vi "ver1(FPGA)_7_8_2013.vi"() -> ()   [LabVIEW 2012]
uses:
  <vilib>/Platform/TimedLoop/XDataNode/timing_clust.ctl
  <vilib>/Platform/TimedLoop/XDataNode/nitl_modes.ctl
  <vilib>/Platform/TimedLoop/XDataNode/wakeup.ctl
  <vilib>/rvi/eio/common/nirviEmuTemplateMethod_errors.vi
  <vilib>/rvi/Emulation/niFpgaSctlEmulationRegisterWithScheduler.vi
  <vilib>/rvi/Emulation/niFpgaSctlEmulationScheduler.vi
  <vilib>/Platform/TimedLoop/XDataNode/XDataNode.xnode
  <vilib>/eio/EIONode/EIONode.xnode
  <vilib>/Platform/TimedLoop/XDataNode/XDNodeRunTimeDep.lvlib
panel:
  in  "Output":bool
  in  "Low Mass Limit":i64
  in  "High Mass Limit":i64
  out "Filter 1 Detector 1 Correlation":i32
  out "Filter 1 Detector 3 Correlation":i32
  out "Velocity Count 1":i32
  in  "Filter 2 threshold":i32=1000
  out "Filter 2 Detector 1 Correlation":i32
  out "Filter 2 Detector 3 Correlation":i32
  out "Velocity Count 2":i32
  in  "Filter 1 threshold":i32=1000
  in  "Filter 3 threshold":i32=1000
  out "Filter 3 Detector 1 Correlation":i32
  out "Filter 3 Detector 3 Correlation":i32
  out "Velocity Count 3":i32
  in  "Filter 4 threshold":i32=1000
  out "Filter 4 Detector 1 Correlation":i32
  out "Filter 4 Detector 3 Correlation":i32
  out "Velocity Count 4":i32
  in  "Filter 5 threshold":i32
  out "Filter 5 Detector 1 Correlation":i32
  out "Filter 5 Detector 3 Correlation":i32
  out "Velocity Count 5":i32
  in  "Filter 6 threshold":i32
  out "Filter 6 Detector 1 Correlation":i32
  out "Filter 6 Detector 3 Correlation":i32
  out "Velocity Count 6":i32
  in  "Filter 7 threshold":i32
  out "Filter 7 Detector 1 Correlation":i32
  out "Filter 7 Detector 3 Correlation":i32
  out "Velocity Count 7":i32
  in  "Noise Level":i32
  out "High Correlation 1":i32
  out "High Correlation 2":i32
  out "High Correlation 3":i32
  out "High Correlation 4":i32
  out "High Correlation 5":i32
  out "High Correlation 6":i32
  out "High Correlation 7":i32
  out "Measured Charge 1":i32
  out "Measured Charge 2":i32
  out "Measured Charge 3":i32
  out "Measured Charge 4":i32
  out "Measured Charge 5":i32
  out "Measured Charge 6":i32
  out "Measured Charge 7":i32
  out "Average 1":i32
  out "Average 2":i32
  out "Average 3":i32
  out "Average 4":i32
  out "Average 5":i32
  out "Average 6":i32
  out "Average 7":i32
  out "Average Out":i32
  in  "Reset Measured Quantities":bool
  out "High Average":i32
  out "High Sample":i32
  out "High Sample I16":i16
  out "Current State 1":u16
  out "Current State 2":u16
  out "Current State 3":u16
  out "Current State 4":u16
  out "Current State 5":u16
  out "Current State 6":u16
  out "Current State 7":u16
  out "Counter 1":i32
  out "Counter 2":i32
  out "Counter 3":i32
  out "Counter 4":i32
  out "Counter 5":i32
  out "Counter 6":i32
  out "Counter 7":i32
  out "Plates":bool
  in  "High Charge Limit":i16
  in  "Low Charge Limit":i16
  in  "High Velocity Count":i32
  in  "Low Velocity Count":i32
  out "Measured Velocity 1":i32
  out "Measured Velocity 2":i32
  out "Measured Velocity 3":i32
  out "Measured Velocity 4":i32
  out "Measured Velocity 5":i32
  out "Measured Velocity 6":i32
  out "Measured Velocity 7":i32
  out "Numeric":i32
  out "IO Module\\AI 0":i16
  out "IO Module\\AI 1":i16
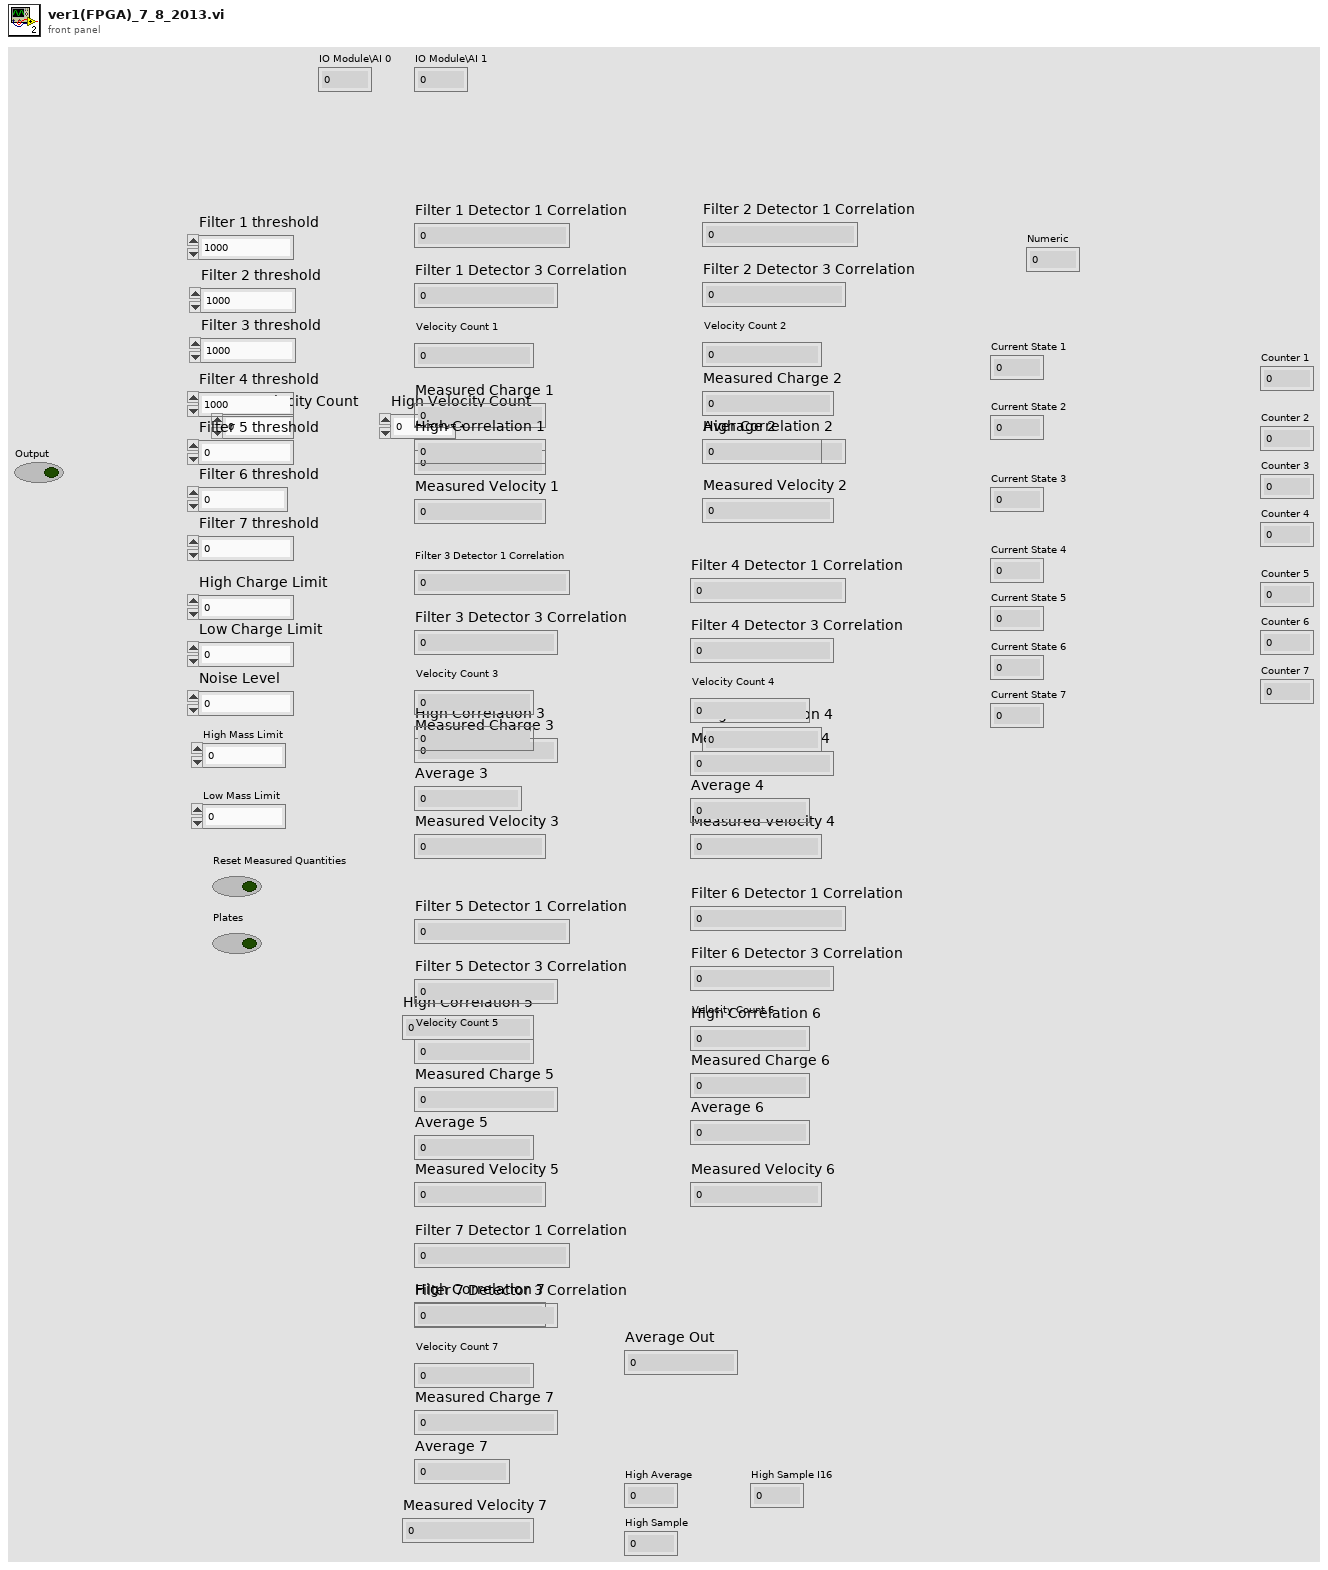
[diagram p1: front panel]
types:
  T1 = typedef "XDNodeRunTimeDep.lvlib/timing_clust.ctl" = cluster{"Expected End [f-1]":u64, "Actual End [f-1]":u64, "Finished Late? [f-1]":bool, "Expected End [i-1]":u64, "Actual End [i-1]":u64, "Finished Late? [i-1]":bool, "Expected Start [i]":u64, "Actual Start [i]":u64, "Expected Start [f]":u64, "Actual Start [f]":u64, "Source Name":string, "Structure Name":string, "Period":i64, "Deadline":i64, "Offset":i64, "Start":i64, "Priority":i32, "Timeout":i32, "Mode":T2, "Wakeup Reason":T3, "Error":errorcluster, "Source Type":string, "Secondary Source Type":string, "Global End Time":u64, "Global Start Time":u64, "Frame Duration":u64, "Iteration Duration":u64, "Assigned CPU":i32, "I/O Scan Engine Mode":u32}
  T2 = typedef "XDNodeRunTimeDep.lvlib/nitl_modes.ctl" = enum32{"No Change", "Process missed periods, maintain original phase", "Discard missed periods, maintain original phase", "Process missed periods, ignore original phase", "Discard missed periods, ignore original phase"}
  T3 = typedef "XDNodeRunTimeDep.lvlib/wakeup.ctl" = enum32{"Normal", "Aborted", "Asynchronous wakeup", "Timing source error", "Timed loop error", "Timeout"}
  T4 = cluster{"Old Average":i32, "New Average":i32, "Current State":u8, "Detector 1 Correlation":i32, "Detector 3 Correlation":i32, "Velocity Count":i32, "Detector Counter in":i32, "Timeout Count in":i32, "Noise Level":i32, "Measured Charge in":i32, "Filter Threshold":i32, "High Correlation in":i32, "Offset":i32, "Offset Average":i32, "Measured Velocity In":i32}
  T5 = cluster{"Separation cut off 1":i32, "Filter Number":i32, "Separation cut off 2":i32}
  T6 = cluster{"High Charge Limit":i16, "Low Charge Limit":i16, "Low Velocity Count":i32, "High Velocity Count":i32, "Low Velocity Count":i32, fxp<+,30,25>, "High Mass Limit":i64, "Low Mass Limit":i64}
  T7 = cluster{"Average Out":i32, "Next State":u8, "Velocity Count out":i32, "Detector counter out":i32, "Timeout count out":u32, "Measured Charge Out":i32, "High Correlation Out":i32, "Plates":bool, "Offset Out":i32, "Measured Velocity Out":i32}
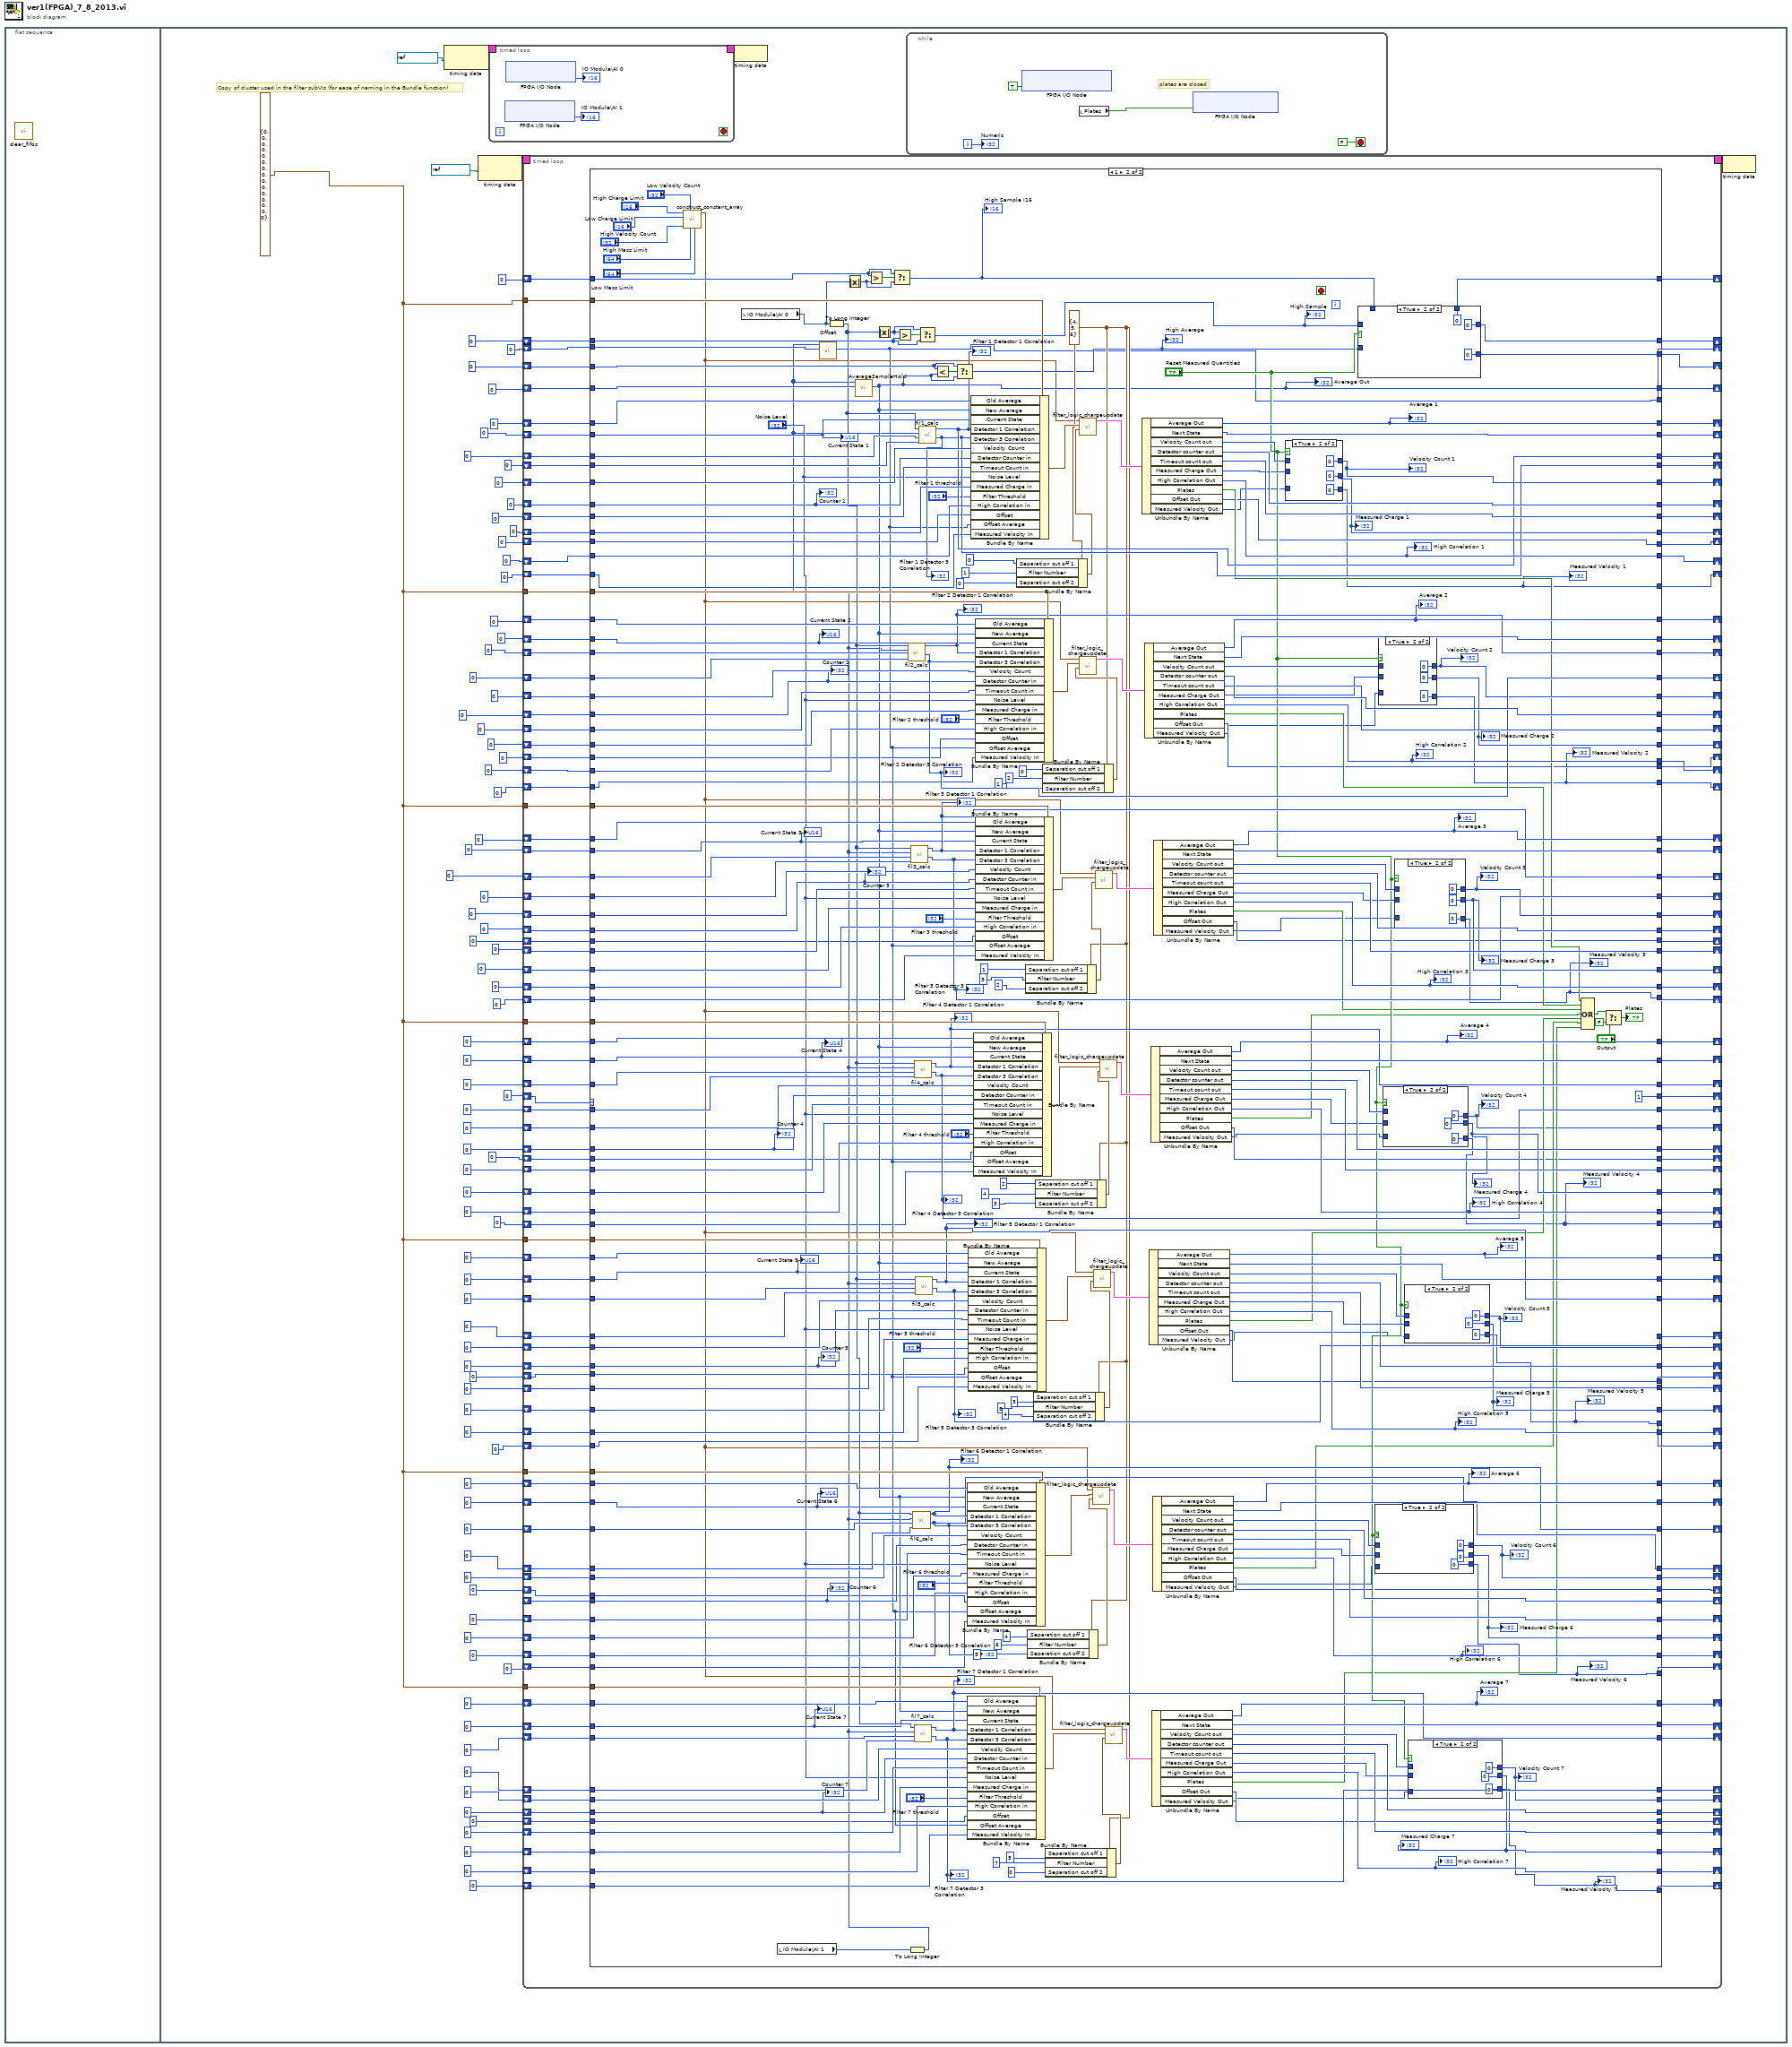
[diagram p0: block diagram]
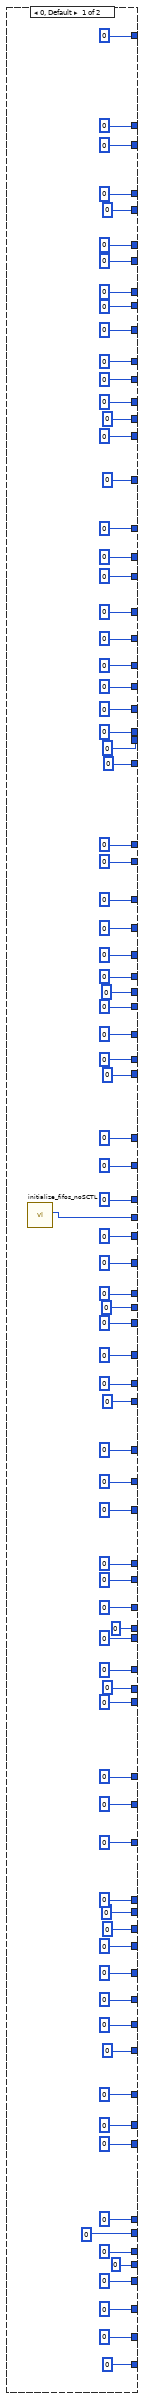
[diagram p2: hidden frame]
diagram:
  n1 = flat-sequence {
    frame #0 {
      n2 = call "clear_fifos.vi"() -> ()  [unwired: 1 in]
    }
    frame #1 {
      w10 = T4 {"Old Average"=0, "New Average"=0, "Current State"=0, "Detector 1 Correlation"=0, "Detector 3 Correlation"=0, "Velocity Count"=0, "Detector Counter in"=0, "Timeout Count in"=0, "Noise Level"=0, "Measured Charge in"=0, "Filter Threshold"=0, "High Correlation in"=0, "Offset"=0, "Offset Average"=0, "Measured Velocity In"=0} ("Variables Cluster")
      # "Copy of cluster used in the filter subVIs (for ease of naming in the Bundle function)"
      n3 = node-c288(refnum<k21> "AI Clock" ("Source Name")) -> (w21:T1)
      n4 = node-c288(refnum<k21> "26 MHz" ("Source Name")) -> (w89:T1)
      n5 = timed-loop {
        timing: w21 -> [_]
        timing-out: [_] -> w20
        stop <- _ stop-if-true
        n6 = xnode "FPGA I/O Node"() -> ("IO Module\\AI 1"=→"IO Module\\AI 1":i16)  [unwired: 1 in, 1 out]
        n7 = xnode "FPGA I/O Node"() -> ("IO Module\\AI 0"=→"IO Module\\AI 0":i16)  [unwired: 1 in, 1 out]
      }
      n8 = timed-loop {
        timing: w89 -> [_]
        timing-out: [_] -> w88
        shift-right: [w267] -> _
        shift-left: 0 ("Velocity Count out") -> [w189]
        shift-right: [w268] -> _
        shift-left: 0 ("Detector 1 Correlation out") -> [w190]
        shift-right: [w154] -> _
        shift-left: 0 ("Detector counter out") -> [w191]
        shift-right: [w185] -> _
        shift-left: 0 ("Next State") -> [w192]
        shift-right: [w153] -> _
        shift-left: 0 ("Detector 3 Correlation out") -> [w188]
        shift-right: [w266] -> _
        shift-left: 0 ("Timeout count out") -> [w187]
        shift-right: [w181] -> _
        shift-left: 0 ("Next State") -> [w184]
        shift-right: [w180] -> _
        shift-left: 0 ("Detector counter out") -> [w183]
        shift-right: [w152] -> _
        shift-left: 0 ("Detector 1 Correlation out") -> [w260]
        shift-right: [w257] -> _
        shift-left: 0 ("Velocity Count out") -> [w259]
        shift-right: [w256] -> _
        shift-left: u32 0 ("Detector 3 Correlation out") -> [w258]
        shift-right: [w251] -> _
        shift-left: 0 ("Timeout count out") -> [w252]
        shift-right: [w175] -> _
        shift-left: 0 ("Next State") -> [w178]
        shift-right: [w150] -> _
        shift-left: 0 ("Detector counter out") -> [w248]
        shift-right: [w246] -> _
        shift-left: 0 ("Detector 1 Correlation out") -> [w247]
        shift-right: [w244] -> _
        shift-left: u32 0 ("Velocity Count out") -> [w245]
        shift-right: [w149] -> _
        shift-left: 0 ("Detector 3 Correlation out") -> [w243]
        shift-right: [w242] -> _
        shift-left: 0 ("Timeout count out") -> [w177]
        shift-right: [w269] -> _
        shift-left: u8 0 ("High Correlation Out") -> [w272]
        shift-right: [w261] -> _
        shift-left: u8 0 ("High Correlation Out") -> [w262]
        shift-right: [w176] -> _
        shift-left: 0 ("High Correlation Out") -> [w179]
        shift-right: [w270] -> _
        shift-left: 0 ("Measured Charge Out") -> [w273]
        shift-right: [w263] -> _
        shift-left: 0 ("Measured Charge Out") -> [w264]
        shift-right: [w250] -> _
        shift-left: u8 0 ("Measured Charge Out") -> [w249]
        shift-right: [w138] -> _
        shift-left: 0 ("Output New Average") -> [w274]
        shift-right: [w186] -> _
        shift-left: 0 ("Detector 1 Correlation Out") -> [w193]
        tunnel: w10 -> [w271]
        shift-right: [w151] -> _
        shift-left: 0 ("High Sample Out") -> [w254]
        shift-right: [w255] -> _
        shift-left: 0 ("High Correlation Out") -> [w182]
        tunnel: w10 -> [w265]
        tunnel: w10 -> [w253]
        shift-right: [w241] -> _
        shift-left: 0 ("Average Out") -> [w240]
        shift-right: [w239] -> _
        shift-left: u8 0 ("Next State") -> [w238]
        shift-right: [w171] -> _
        shift-left: 0 ("Detector 1 Correlation out") -> [w173]
        shift-right: [w170] -> _
        shift-left: 0 ("Detector 3 Correlation out") -> [w172]
        shift-right: [w148] -> _
        shift-left: 0 ("Velocity Count out") -> [w237]
        shift-right: [w236] -> _
        shift-left: 0 ("Detector counter out") -> [w235]
        shift-right: [w234] -> _
        shift-left: u32 0 ("Timeout count out") -> [w233]
        shift-right: [w147] -> _
        shift-left: 0 ("Measured Charge Out") -> [w232]
        shift-right: [w231] -> _
        shift-left: 0 ("High Correlation Out") -> [w174]
        tunnel: w10 -> [w230]
        shift-right: [w228] -> _
        shift-left: 0 ("Average Out") -> [w227]
        shift-right: [w226] -> _
        shift-left: u8 0 ("Next State") -> [w225]
        shift-right: [w166] -> _
        shift-left: 0 ("Detector 1 Correlation out") -> [w169]
        shift-right: [w165] -> _
        shift-left: 0 ("Detector 3 Correlation out") -> [w168]
        shift-right: [w146] -> _
        shift-left: 0 ("Velocity Count out") -> [w224]
        shift-right: [w223] -> _
        shift-left: 0 ("Detector counter out") -> [w222]
        shift-right: [w221] -> _
        shift-left: u32 0 ("Timeout count out") -> [w220]
        shift-right: [w145] -> _
        shift-left: 0 ("Measured Charge Out") -> [w219]
        shift-right: [w218] -> _
        shift-left: 0 ("High Correlation Out") -> [w167]
        tunnel: w10 -> [w229]
        shift-right: [w216] -> _
        shift-left: 0 ("Average Out") -> [w214]
        shift-right: [w215] -> _
        shift-left: u8 0 ("Next State") -> [w211]
        shift-right: [w161] -> _
        shift-left: 0 ("Detector 1 Correlation out") -> [w164]
        shift-right: [w160] -> _
        shift-left: 0 ("Detector 3 Correlation out") -> [w163]
        shift-right: [w143] -> _
        shift-left: 0 ("Velocity Count out") -> [w213]
        shift-right: [w210] -> _
        shift-left: _ -> [w212]
        shift-right: [w209] -> _
        shift-left: u32 0 ("Timeout count out") -> [w208]
        shift-right: [w144] -> _
        shift-left: 0 ("Measured Charge Out") -> [w207]
        shift-right: [w206] -> _
        shift-left: 0 ("High Correlation Out") -> [w162]
        tunnel: w10 -> [w217]
        shift-right: [w204] -> _
        shift-left: 0 ("Average Out") -> [w203]
        shift-right: [w202] -> _
        shift-left: u8 0 ("Next State") -> [w194]
        shift-right: [w156] -> _
        shift-left: 0 ("Detector 1 Correlation out") -> [w159]
        shift-right: [w155] -> _
        shift-left: 0 ("Detector 3 Correlation out") -> [w158]
        shift-right: [w142] -> _
        shift-left: 0 ("Velocity Count out") -> [w201]
        shift-right: [w200] -> _
        shift-left: 0 ("Detector counter out") -> [w199]
        shift-right: [w198] -> _
        shift-left: u32 0 ("Timeout count out") -> [w197]
        shift-right: [w141] -> _
        shift-left: 0 ("Measured Charge Out") -> [w196]
        shift-right: [w195] -> _
        shift-left: 0 ("High Correlation Out") -> [w157]
        tunnel: w10 -> [w205]
        shift-right: [w136] -> _
        shift-left: 0 -> [w137]
        shift-right: [w139] -> _
        shift-left: 0 -> [w140]
        shift-right: [w134] -> _
        shift-left: i16 0 -> [w135]
        shift-right: [w132] -> _
        shift-left: i16 0 -> [w133]
        shift-right: [w130] -> _
        shift-left: 0 -> [w131]
        shift-right: [w129] -> _
        shift-left: 0 -> [w126]
        shift-right: [w127] -> _
        shift-left: 0 -> [w128]
        shift-right: [w124] -> _
        shift-left: 0 ("Offset Out") -> [w125]
        shift-right: [w123] -> _
        shift-left: 0 ("Offset Out") -> [w122]
        shift-right: [w121] -> _
        shift-left: 0 ("Offset Out") -> [w120]
        shift-right: [w119] -> _
        shift-left: 0 ("Offset Out") -> [w118]
        shift-right: [w117] -> _
        shift-left: 0 ("Offset Out") -> [w116]
        shift-right: [w114] -> _
        shift-left: 0 -> [w115]
        shift-right: [w113] -> _
        shift-left: 0 -> [w102]
        shift-right: [w112] -> _
        shift-left: 0 -> [w103]
        shift-right: [w111] -> _
        shift-left: 0 -> [w104]
        shift-right: [w110] -> _
        shift-left: 0 -> [w105]
        shift-right: [w109] -> _
        shift-left: 0 -> [w106]
        shift-right: [w108] -> _
        shift-left: 0 ("Measured Velocity Out") -> [w107]
        stop <- _ stop-if-true
        n9 = case shown="1" w133 {
          tunnel: w274 -> [_ w632]
          tunnel: w273 -> [_ w631]
          tunnel: w272 -> [_ w424]
          tunnel: w271 -> [_ w630]
          tunnel: [0 ("Average Out") w629] -> w270
          tunnel: [u16 0 ("Next State") w628] -> w269
          tunnel: [0 ("Detector counter out") w627] -> w268
          tunnel: [u32 0 ("Timeout count out") w626] -> w267
          tunnel: [0 ("High Correlation Out") w625] -> w266
          tunnel: w265 -> [_ w624]
          tunnel: w264 -> [_ w623]
          tunnel: [0 ("Average Out") w622] -> w263
          tunnel: w262 -> [_ w423]
          tunnel: [u16 0 ("Next State") w621] -> w261
          tunnel: w260 -> [_ w620]
          tunnel: w259 -> [_ w416]
          tunnel: w258 -> [_ w619]
          tunnel: [0 ("Detector counter out") w618] -> w257
          tunnel: [u32 0 ("Timeout count out") w617] -> w256
          tunnel: [0 ("High Correlation Out") w616] -> w255
          tunnel: w254 -> [_ w615]
          tunnel: w253 -> [_ w614]
          tunnel: w252 -> [_ w613]
          tunnel: [0 ("Average Out") w612] -> w251
          tunnel: [u16 0 ("Next State") w611] -> w250
          tunnel: w249 -> [_ w422]
          tunnel: w248 -> [_ w610]
          tunnel: w247 -> [_ w415]
          tunnel: [0 ("Detector counter out") w609] -> w246
          tunnel: w245 -> [_ w608]
          tunnel: [u32 0 ("Timeout count out") w607] -> w244
          tunnel: w243 -> [_ w606]
          tunnel: [0 ("High Correlation Out") w605] -> w242
          tunnel: [0 ("Average Out") w604] -> w241
          tunnel: w240 -> [_ w603]
          tunnel: [u16 0 ("Next State") w602] -> w239
          tunnel: w238 -> [_ w421]
          tunnel: w237 -> [_ w601]
          tunnel: [0 ("Detector counter out") w600] -> w236
          tunnel: w235 -> [_ w414]
          tunnel: [u32 0 ("Timeout count out") w599] -> w234
          tunnel: w233 -> [_ w598]
          tunnel: w232 -> [_ w597]
          tunnel: [0 ("High Correlation Out") w596] -> w231
          tunnel: w230 -> [_ w595]
          tunnel: w229 -> [_ w594]
          tunnel: [0 ("Average Out") w593] -> w228
          tunnel: w227 -> [_ w592]
          tunnel: [u16 0 ("Next State") w591] -> w226
          tunnel: w225 -> [_ w420]
          tunnel: w224 -> [_ w590]
          tunnel: [0 ("Detector counter out") w589] -> w223
          tunnel: w222 -> [_ w413]
          tunnel: [u32 0 ("Timeout count out") w588] -> w221
          tunnel: w220 -> [_ w587]
          tunnel: w219 -> [_ w586]
          tunnel: [0 ("High Correlation Out") w585] -> w218
          tunnel: w217 -> [_ w584]
          tunnel: [0 ("Average Out") w583] -> w216
          tunnel: [u16 0 ("Next State") w582] -> w215
          tunnel: w214 -> [_ w581]
          tunnel: w213 -> [_ w580]
          tunnel: w212 -> [_ w412]
          tunnel: w211 -> [_ w419]
          tunnel: [0 ("Detector counter out") w579] -> w210
          tunnel: [u32 0 ("Timeout count out") w578] -> w209
          tunnel: w208 -> [_ w577]
          tunnel: w207 -> [_ w576]
          tunnel: [0 ("High Correlation Out") w575] -> w206
          tunnel: w205 -> [_ w574]
          tunnel: [0 ("Average Out") w573] -> w204
          tunnel: w203 -> [_ w572]
          tunnel: [u16 0 ("Next State") w571] -> w202
          tunnel: w201 -> [_ w570]
          tunnel: [0 ("Detector counter out") w569] -> w200
          tunnel: w199 -> [_ w411]
          tunnel: [u32 0 ("Timeout count out") w568] -> w198
          tunnel: w197 -> [_ w567]
          tunnel: w196 -> [_ w566]
          tunnel: [0 ("High Correlation Out") w565] -> w195
          tunnel: w194 -> [_ w418]
          tunnel: w193 -> [_ w564]
          tunnel: w192 -> [_ w563]
          tunnel: w191 -> [_ w562]
          tunnel: w190 -> [_ w417]
          tunnel: w189 -> [_ w561]
          tunnel: w188 -> [_ w560]
          tunnel: w187 -> [_ w559]
          tunnel: [0 ("Detector 1 Correlation Out") w558] -> w186
          tunnel: [0 ("Detector 3 Correlation Out") w557] -> w185
          tunnel: w184 -> [_ w556]
          tunnel: w183 -> [_ w555]
          tunnel: w182 -> [_ w554]
          tunnel: [0 ("Detector 1 Correlation Out") w553] -> w181
          tunnel: [0 ("Detector 3 Correlation Out") w552] -> w180
          tunnel: w179 -> [_ w551]
          tunnel: w178 -> [_ w550]
          tunnel: w177 -> [_ w549]
          tunnel: [0 ("Detector 1 Correlation Out") w548] -> w176
          tunnel: [0 ("Detector 3 Correlation Out") w547] -> w175
          tunnel: w174 -> [_ w546]
          tunnel: w173 -> [_ w545]
          tunnel: w172 -> [_ w544]
          tunnel: [0 ("Detector 1 Correlation Out") w543] -> w171
          tunnel: [0 ("Detector 3 Correlation Out") w542] -> w170
          tunnel: w169 -> [_ w541]
          tunnel: w168 -> [_ w540]
          tunnel: w167 -> [_ w539]
          tunnel: [0 ("Detector 1 Correlation Out") w538] -> w166
          tunnel: [0 ("Detector 3 Correlation Out") w537] -> w165
          tunnel: w164 -> [_ w536]
          tunnel: w163 -> [_ w535]
          tunnel: w162 -> [_ w534]
          tunnel: [0 ("Detector 1 Correlation Out") w533] -> w161
          tunnel: [0 ("Detector 3 Correlation Out") w532] -> w160
          tunnel: w159 -> [_ w531]
          tunnel: w158 -> [_ w530]
          tunnel: w157 -> [_ w529]
          tunnel: [0 ("Detector 1 Correlation Out") w528] -> w156
          tunnel: [0 ("Detector 3 Correlation Out") w527] -> w155
          tunnel: [0 ("Velocity Count out") w526] -> w154
          tunnel: [0 ("Measured Charge Out") w525] -> w153
          tunnel: [0 ("Velocity Count out") w524] -> w152
          tunnel: [0 ("Measured Charge Out") w523] -> w151
          tunnel: [0 ("Velocity Count out") w522] -> w150
          tunnel: [0 ("Measured Charge Out") w521] -> w149
          tunnel: [0 ("Velocity Count out") w410] -> w148
          tunnel: [0 ("Measured Charge Out") w520] -> w147
          tunnel: [0 ("Velocity Count out") w519] -> w146
          tunnel: [0 ("Measured Charge Out") w518] -> w145
          tunnel: [0 ("Measured Charge Out") w517] -> w144
          tunnel: [0 ("Velocity Count out") w516] -> w143
          tunnel: [0 ("Velocity Count out") w515] -> w142
          tunnel: [0 ("Measured Charge Out") w514] -> w141
          tunnel: w140 -> [_ w513]
          tunnel: [0 w512] -> w139
          tunnel: [0 ("Output New Average") w409] -> w138
          tunnel: w137 -> [_ w511]
          tunnel: [0 w510] -> w136
          tunnel: w135 -> [_ w509]
          tunnel: [i16 0 w508] -> w134
          tunnel: [w357 i16 1 ("Output State")] -> w132
          tunnel: w131 -> [_ w406]
          tunnel: [0 ("Offset Out") w405] -> w130
          tunnel: [0 ("Offset Out") w404] -> w129
          tunnel: w128 -> [_ w403]
          tunnel: [0 ("Output New Average") w392] -> w127
          tunnel: w126 -> [_ w401]
          tunnel: w125 -> [_ w400]
          tunnel: [0 ("Offset Out") w399] -> w124
          tunnel: [0 ("Offset Out") w398] -> w123
          tunnel: w122 -> [_ w397]
          tunnel: [0 ("Offset Out") w396] -> w121
          tunnel: w120 -> [_ w395]
          tunnel: [0 ("Offset Out") w394] -> w119
          tunnel: w118 -> [_ w393]
          tunnel: [0 ("Offset Out") w391] -> w117
          tunnel: w116 -> [_ w390]
          tunnel: w115 -> [_ w385]
          tunnel: [0 ("Measured Velocity Out") w377] -> w114
          tunnel: [0 ("Measured Velocity Out") w375] -> w113
          tunnel: [0 ("Measured Velocity Out") w373] -> w112
          tunnel: [0 ("Measured Velocity Out") w371] -> w111
          tunnel: [0 ("Measured Velocity Out") w369] -> w110
          tunnel: [0 ("Measured Velocity Out") w367] -> w109
          tunnel: [0 ("Measured Velocity Out") w365] -> w108
          tunnel: w107 -> [_ w384]
          tunnel: w106 -> [_ w383]
          tunnel: w105 -> [_ w382]
          tunnel: w104 -> [_ w381]
          tunnel: w103 -> [_ w380]
          tunnel: w102 -> [_ w379]
          frame 0, Default {
            n10 = call "initialize_fifos_noSCTL.vi"() -> ("Output State"=w357:i16)  [unwired: 11 in]
          }
          frame 1 {
            w460 = T5 {"Separation cut off 1"=4, "Filter Number"=5, "Separation cut off 2"=6} ("Filter Specific Constants")
            n11 = call "construct_constant_array.vi"("Low Mass Limit"="Low Mass Limit", "High Mass Limit"="High Mass Limit", "Low Velocity Count"="Low Velocity Count", "High Velocity Count"="High Velocity Count", "Low Charge Limit"="Low Charge Limit", "High Charge Limit"="High Charge Limit") -> ("constants cluster"=w362:T6)  [unwired: 5 in]
            n12 = local read "IO Module\\AI 0"() -> (w408:i16)
            n13 = local read "IO Module\\AI 1"() -> (w407:i16)
            n14 = To Long Integer(number=w408) -> (32bit integer=w441:i32)
            n15 = Absolute Value(x=w408) -> (abs(x)=w434:i16)
            n16 = Greater?(x=w509, y=w434) -> (0:w435:bool)
            n17 = Absolute Value(x=w441) -> (abs(x)=w439:i32)
            n18 = Select(t=w509, s=w435, f=w434) -> (s? t:f=w433:i16)
            "High Sample I16" <- w433
            n19 = Greater?(x=w439, y=w513) -> (0:w440:bool)
            n20 = To Long Integer(number=w407) -> (32bit integer=w402:i32)
            n21 = call "Offset.vi"("Previous Average"=w403, "Input Value"=w402) -> ("Output New Average"=w392:i32)  [unwired: 7 in]
            n22 = call "AverageSampleHold.vi"("Previous Average"=w632, "Input Value"=w402) -> ("Output New Average"=w409:i32)  [unwired: 7 in]
            "Average Out" <- w409
            n23 = call "fil2_calc.vi"("Detector 3 Correlation In"=w555, "Detector 1 Correlation In"=w556, "AI1"=w402, "AI0"=w441) -> ("Detector 3 Correlation Out"=w552:i32, "Detector 1 Correlation Out"=w553:i32)  [unwired: 4 in]
            "Filter 2 Detector 1 Correlation" <- w553
            "Filter 2 Detector 3 Correlation" <- w552
            n24 = call "fil3_calc.vi"("Detector 3 Correlation In"=w550, "Detector 1 Correlation In"=w551, "AI1"=w402, "AI0"=w441) -> ("Detector 3 Correlation Out"=w547:i32, "Detector 1 Correlation Out"=w548:i32)  [unwired: 4 in]
            "Filter 3 Detector 1 Correlation" <- w548
            "Filter 3 Detector 3 Correlation" <- w547
            n25 = call "fil6_calc.vi"("Detector 3 Correlation In"=w535, "Detector 1 Correlation In"=w536, "AI1"=w402, "AI0"=w441) -> ("Detector 3 Correlation Out"=w532:i32, "Detector 1 Correlation Out"=w533:i32)  [unwired: 4 in]
            "Filter 6 Detector 1 Correlation" <- w533
            "Filter 6 Detector 3 Correlation" <- w532
            n26 = call "fil4_calc.vi"("Detector 3 Correlation In"=w544, "Detector 1 Correlation In"=w545, "AI1"=w402, "AI0"=w441) -> ("Detector 3 Correlation Out"=w542:i32, "Detector 1 Correlation Out"=w543:i32)  [unwired: 4 in]
            "Filter 4 Detector 1 Correlation" <- w543
            "Filter 4 Detector 3 Correlation" <- w542
            n27 = call "fil7_calc.vi"("Detector 3 Correlation In"=w530, "Detector 1 Correlation In"=w531, "AI1"=w402, "AI0"=w441) -> ("Detector 3 Correlation Out"=w527:i32, "Detector 1 Correlation Out"=w528:i32)  [unwired: 4 in]
            "Filter 7 Detector 1 Correlation" <- w528
            "Filter 7 Detector 3 Correlation" <- w527
            n28 = call "fil5_calc.vi"("Detector 3 Correlation In"=w540, "Detector 1 Correlation In"=w541, "AI1"=w402, "AI0"=w441) -> ("Detector 3 Correlation Out"=w537:i32, "Detector 1 Correlation Out"=w538:i32)  [unwired: 4 in]
            "Filter 5 Detector 1 Correlation" <- w538
            "Filter 5 Detector 3 Correlation" <- w537
            n29 = call "fil1_calc.vi"("Detector 3 Correlation In"=w563, "Detector 1 Correlation In"=w564, "AI1"=w402, "AI0"=w441) -> ("Detector 3 Correlation Out"=w557:i32, "Detector 1 Correlation Out"=w558:i32)  [unwired: 4 in]
            "Filter 1 Detector 1 Correlation" <- w558
            "Filter 1 Detector 3 Correlation" <- w557
            n30 = Select(t=w439, s=w440, f=w513) -> (s? t:f=w436:i32)
            "High Sample" <- w436
            n31 = Less?(x=w511, y=w409) -> (x < y?=w438:bool)
            n32 = Select(t=w511, s=w438, f=w409) -> (s? t:f=w437:i32)
            "High Average" <- w437
            n33 = Bundle By Name(cluster=w584, "Old Average"=w581, "New Average"=w409, "Current State"=w419, "Detector 1 Correlation"=w533, "Detector 3 Correlation"=w532, "Velocity Count"=w580, "Detector Counter in"=w412, "Timeout Count in"=w577, "Noise Level"="Noise Level", "Measured Charge in"=w576, "Filter Threshold"="Filter 6 threshold", "High Correlation in"=w534, "Offset"=w393, "Offset Average"=w392, "Measured Velocity In"=w383) -> (w482:T4)
            n34 = Bundle By Name(cluster=w574, "Old Average"=w572, "New Average"=w409, "Current State"=w418, "Detector 1 Correlation"=w528, "Detector 3 Correlation"=w527, "Velocity Count"=w570, "Detector Counter in"=w411, "Timeout Count in"=w567, "Noise Level"="Noise Level", "Measured Charge in"=w566, "Filter Threshold"="Filter 7 threshold", "High Correlation in"=w529, "Offset"=w390, "Offset Average"=w392, "Measured Velocity In"=w384) -> (w497:T4)
            n35 = Bundle By Name(cluster=w594, "Old Average"=w592, "New Average"=w409, "Current State"=w420, "Detector 1 Correlation"=w538, "Detector 3 Correlation"=w537, "Velocity Count"=w590, "Detector Counter in"=w413, "Timeout Count in"=w587, "Noise Level"="Noise Level", "Measured Charge in"=w586, "Filter Threshold"="Filter 5 threshold", "High Correlation in"=w539, "Offset"=w395, "Offset Average"=w392, "Measured Velocity In"=w382) -> (w485:T4)
            n36 = Bundle By Name(cluster=w630, "Old Average"=w631, "New Average"=w409, "Current State"=w424, "Detector 1 Correlation"=w558, "Detector 3 Correlation"=w557, "Velocity Count"=w562, "Detector Counter in"=w417, "Timeout Count in"=w561, "Noise Level"="Noise Level", "Measured Charge in"=w560, "Filter Threshold"="Filter 1 threshold", "High Correlation in"=w559, "Offset"=w406, "Offset Average"=w392, "Measured Velocity In"=w385) -> (w494:T4)
            n37 = Bundle By Name(cluster=w595, "Old Average"=w603, "New Average"=w409, "Current State"=w421, "Detector 1 Correlation"=w543, "Detector 3 Correlation"=w542, "Velocity Count"=w601, "Detector Counter in"=w414, "Timeout Count in"=w598, "Noise Level"="Noise Level", "Measured Charge in"=w597, "Filter Threshold"="Filter 4 threshold", "High Correlation in"=w546, "Offset"=w397, "Offset Average"=w392, "Measured Velocity In"=w381) -> (w488:T4)
            n38 = Bundle By Name(cluster=w624, "Old Average"=w623, "New Average"=w409, "Current State"=w423, "Detector 1 Correlation"=w553, "Detector 3 Correlation"=w552, "Velocity Count"=w620, "Detector Counter in"=w416, "Timeout Count in"=w619, "Noise Level"="Noise Level", "Measured Charge in"=w615, "Filter Threshold"="Filter 2 threshold", "High Correlation in"=w554, "Offset"=w401, "Offset Average"=w392, "Measured Velocity In"=w379) -> (w506:T4)
            n39 = Bundle By Name(cluster=w614, "Old Average"=w613, "New Average"=w409, "Current State"=w422, "Detector 1 Correlation"=w548, "Detector 3 Correlation"=w547, "Velocity Count"=w610, "Detector Counter in"=w415, "Timeout Count in"=w608, "Noise Level"="Noise Level", "Measured Charge in"=w606, "Filter Threshold"="Filter 3 threshold", "High Correlation in"=w549, "Offset"=w400, "Offset Average"=w392, "Measured Velocity In"=w380) -> (w491:T4)
            n40 = Bundle By Name(cluster=w460, "Separation cut off 1"=0, "Filter Number"=1, "Separation cut off 2"=0) -> (w493:T5)
            n41 = Bundle By Name(cluster=w460, "Separation cut off 1"=1, "Filter Number"=3, "Separation cut off 2"=2) -> (w490:T5)
            n42 = Bundle By Name(cluster=w460, "Separation cut off 1"=4, "Filter Number"=6, "Separation cut off 2"=5) -> (w481:T5)
            n43 = Bundle By Name(cluster=w460, "Separation cut off 1"=3, "Filter Number"=5, "Separation cut off 2"=4) -> (w484:T5)
            n44 = Bundle By Name(cluster=w460, "Separation cut off 1"=2, "Filter Number"=4, "Separation cut off 2"=3) -> (w487:T5)
            n45 = Bundle By Name(cluster=w460, "Separation cut off 1"=0, "Filter Number"=2, "Separation cut off 2"=1) -> (w498:T5)
            n46 = Bundle By Name(cluster=w460, "Separation cut off 1"=5, "Filter Number"=7, "Separation cut off 2"=0) -> (w496:T5)
            n47 = call "filter_logic_chargeupdate.vi"("Filter Specific Constants"=w493, "Variables Cluster"=w494, "constants cluster"=w362) -> ("Output Cluster"=w492:T7)  [unwired: 8 in]
            n48 = call "filter_logic_chargeupdate.vi"("Filter Specific Constants"=w498, "Variables Cluster"=w506, "constants cluster"=w362) -> ("Output Cluster"=w505:T7)  [unwired: 8 in]
            n49 = call "filter_logic_chargeupdate.vi"("Filter Specific Constants"=w481, "Variables Cluster"=w482, "constants cluster"=w362) -> ("Output Cluster"=w480:T7)  [unwired: 8 in]
            n50 = call "filter_logic_chargeupdate.vi"("Filter Specific Constants"=w484, "Variables Cluster"=w485, "constants cluster"=w362) -> ("Output Cluster"=w483:T7)  [unwired: 8 in]
            n51 = call "filter_logic_chargeupdate.vi"("Filter Specific Constants"=w490, "Variables Cluster"=w491, "constants cluster"=w362) -> ("Output Cluster"=w489:T7)  [unwired: 8 in]
            n52 = call "filter_logic_chargeupdate.vi"("Filter Specific Constants"=w487, "Variables Cluster"=w488, "constants cluster"=w362) -> ("Output Cluster"=w486:T7)  [unwired: 8 in]
            n53 = call "filter_logic_chargeupdate.vi"("Filter Specific Constants"=w496, "Variables Cluster"=w497, "constants cluster"=w362) -> ("Output Cluster"=w495:T7)  [unwired: 8 in]
            n54 = Unbundle By Name(w492) -> ("Average Out"=w629:i32, "Next State"=w628:u8, "Velocity Count out"=w456:i32, "Detector counter out"=w627:i32, "Timeout count out"=w626:u32, "Measured Charge Out"=w455:i32, "High Correlation Out"=w625:i32, "Plates"=w431:bool, "Offset Out"=w405:i32, "Measured Velocity Out"=w378:i32)
            "High Correlation 1" <- w625
            "Average 1" <- w629
            n55 = Unbundle By Name(w505) -> ("Average Out"=w622:i32, "Next State"=w621:u8, "Velocity Count out"=w454:i32, "Detector counter out"=w618:i32, "Timeout count out"=w617:u32, "Measured Charge Out"=w453:i32, "High Correlation Out"=w616:i32, "Plates"=w430:bool, "Offset Out"=w404:i32, "Measured Velocity Out"=w376:i32)
            "High Correlation 2" <- w616
            "Average 2" <- w622
            n56 = Unbundle By Name(w483) -> ("Average Out"=w593:i32, "Next State"=w591:u8, "Velocity Count out"=w448:i32, "Detector counter out"=w589:i32, "Timeout count out"=w588:u32, "Measured Charge Out"=w447:i32, "High Correlation Out"=w585:i32, "Plates"=w427:bool, "Offset Out"=w396:i32, "Measured Velocity Out"=w370:i32)
            "High Correlation 5" <- w585
            "Average 5" <- w593
            n57 = Unbundle By Name(w486) -> ("Average Out"=w604:i32, "Next State"=w602:u8, "Velocity Count out"=w450:i32, "Detector counter out"=w600:i32, "Timeout count out"=w599:u32, "Measured Charge Out"=w449:i32, "High Correlation Out"=w596:i32, "Plates"=w428:bool, "Offset Out"=w398:i32, "Measured Velocity Out"=w372:i32)
            "High Correlation 4" <- w596
            "Average 4" <- w604
            n58 = Unbundle By Name(w495) -> ("Average Out"=w573:i32, "Next State"=w571:u8, "Velocity Count out"=w444:i32, "Detector counter out"=w569:i32, "Timeout count out"=w568:u32, "Measured Charge Out"=w443:i32, "High Correlation Out"=w565:i32, "Plates"=w425:bool, "Offset Out"=w391:i32, "Measured Velocity Out"=w366:i32)
            "High Correlation 7" <- w565
            "Average 7" <- w573
            n59 = Unbundle By Name(w480) -> ("Average Out"=w583:i32, "Next State"=w582:u8, "Velocity Count out"=w446:i32, "Detector counter out"=w579:i32, "Timeout count out"=w578:u32, "Measured Charge Out"=w445:i32, "High Correlation Out"=w575:i32, "Plates"=w426:bool, "Offset Out"=w394:i32, "Measured Velocity Out"=w368:i32)
            "High Correlation 6" <- w575
            "Average 6" <- w583
            n60 = Unbundle By Name(w489) -> ("Average Out"=w612:i32, "Next State"=w611:u8, "Velocity Count out"=w452:i32, "Detector counter out"=w609:i32, "Timeout count out"=w607:u32, "Measured Charge Out"=w451:i32, "High Correlation Out"=w605:i32, "Plates"=w429:bool, "Offset Out"=w399:i32, "Measured Velocity Out"=w374:i32)
            "High Correlation 3" <- w605
            "Average 3" <- w612
            n61 = case shown="True" "Reset Measured Quantities" {
              tunnel: w456 -> [w677 _]
              tunnel: [w677 0 ("Velocity Count out")] -> w526
              tunnel: w455 -> [w676 _]
              tunnel: [w676 0 ("Measured Charge Out")] -> w525
              tunnel: w378 -> [w675 _]
              tunnel: [w675 0 ("Measured Velocity Out")] -> w377
              frame False {
              }
              frame True {
              }
            }
            "Velocity Count 1" <- w526
            "Measured Charge 1" <- w525
            "Measured Velocity 1" <- w377
            n62 = case shown="True" "Reset Measured Quantities" {
              tunnel: w436 -> [w635 _]
              tunnel: [w635 0] -> w512
              tunnel: w437 -> [w634 _]
              tunnel: [w634 0] -> w510
              tunnel: w433 -> [w633 _]
              tunnel: [w633 i16 0] -> w508
              frame False {
              }
              frame True {
              }
            }
            n63 = case shown="True" "Reset Measured Quantities" {
              tunnel: w446 -> [w647 _]
              tunnel: [w647 0 ("Velocity Count out")] -> w516
              tunnel: w445 -> [w646 _]
              tunnel: [w646 0 ("Measured Charge Out")] -> w517
              tunnel: w368 -> [w645 _]
              tunnel: [w645 0 ("Measured Velocity Out")] -> w367
              frame False {
              }
              frame True {
              }
            }
            "Velocity Count 6" <- w516
            "Measured Charge 6" <- w517
            "Measured Velocity 6" <- w367
            n64 = case shown="True" "Reset Measured Quantities" {
              tunnel: w454 -> [w671 _]
              tunnel: [w671 0 ("Velocity Count out")] -> w524
              tunnel: w453 -> [w670 _]
              tunnel: [w670 0 ("Measured Charge Out")] -> w523
              tunnel: w376 -> [w669 _]
              tunnel: [w669 0 ("Measured Velocity Out")] -> w375
              frame False {
              }
              frame True {
              }
            }
            "Velocity Count 2" <- w524
            "Measured Charge 2" <- w523
            "Measured Velocity 2" <- w375
            n65 = case shown="True" "Reset Measured Quantities" {
              tunnel: w450 -> [w659 _]
              tunnel: [w659 0 ("Velocity Count out")] -> w410
              tunnel: w449 -> [w658 _]
              tunnel: [w658 0 ("Measured Charge Out")] -> w520
              tunnel: w372 -> [w657 _]
              tunnel: [w657 0 ("Measured Velocity Out")] -> w371
              frame False {
              }
              frame True {
              }
            }
            "Velocity Count 4" <- w410
            "Measured Charge 4" <- w520
            "Measured Velocity 4" <- w371
            n66 = case shown="True" "Reset Measured Quantities" {
              tunnel: w452 -> [w665 _]
              tunnel: [w665 0 ("Velocity Count out")] -> w522
              tunnel: w451 -> [w664 _]
              tunnel: [w664 0 ("Measured Charge Out")] -> w521
              tunnel: w374 -> [w663 _]
              tunnel: [w663 0 ("Measured Velocity Out")] -> w373
              frame False {
              }
              frame True {
              }
            }
            "Velocity Count 3" <- w522
            "Measured Charge 3" <- w521
            "Measured Velocity 3" <- w373
            n67 = case shown="True" "Reset Measured Quantities" {
              tunnel: w448 -> [w653 _]
              tunnel: [w653 0 ("Velocity Count out")] -> w519
              tunnel: w447 -> [w652 _]
              tunnel: [w652 0 ("Measured Charge Out")] -> w518
              tunnel: w370 -> [w651 _]
              tunnel: [w651 0 ("Measured Velocity Out")] -> w369
              frame False {
              }
              frame True {
              }
            }
            "Velocity Count 5" <- w519
            "Measured Charge 5" <- w518
            "Measured Velocity 5" <- w369
            n68 = case shown="True" "Reset Measured Quantities" {
              tunnel: w444 -> [w641 _]
              tunnel: [w641 0 ("Velocity Count out")] -> w515
              tunnel: w443 -> [w640 _]
              tunnel: [w640 0 ("Measured Charge Out")] -> w514
              tunnel: w366 -> [w639 _]
              tunnel: [w639 0 ("Measured Velocity Out")] -> w365
              frame False {
              }
              frame True {
              }
            }
            "Velocity Count 7" <- w515
            "Measured Charge 7" <- w514
            "Measured Velocity 7" <- w365
            n69 = Compound Arithmetic op=OR(w431, w430, w429, w428, w427, w426, w425) -> (w361:bool)
            n70 = Select(t=w361, s="Output", f=FALSE) -> (s? t:f=→"Plates":bool)
            "Current State 1" <- w424
            "Current State 2" <- w423
            "Current State 3" <- w422
            "Current State 4" <- w421
            "Current State 5" <- w420
            "Current State 6" <- w419
            "Current State 7" <- w418
            "Counter 1" <- w417
            "Counter 2" <- w416
            "Counter 3" <- w415
            "Counter 4" <- w414
            "Counter 5" <- w413
            "Counter 6" <- w412
            "Counter 7" <- w411
          }
        }
      }
      n71 = node-c288(w20) -> ()
      n72 = while {
        i -> [w101]
        stop <- FALSE stop-if-true
        # "plates are closed"
        n73 = xnode "FPGA I/O Node"("IO Module\\PFI Enable"=TRUE ("IO Module\\PFI Enable")) -> ()  [unwired: 1 in, 1 out]
        n74 = local read "Plates"() -> (w100:bool)
        n75 = xnode "FPGA I/O Node"("IO Module\\PFI Out 4"=w100) -> ()  [unwired: 1 in, 1 out]
        "Numeric" <- w101
      }
      n76 = node-c288(w88) -> ()
    }
  }
